vi "Init.vi"(8 "error in (no error)":errorcluster, 9 "Minimum Event Level":T1=enum."Info", 10 "EventLogger":refnum<class "EventLogHandler.lvclass">) -> (0 "error out":errorcluster, 3 "EventLoggingService out":refnum<class "EventLoggingService.lvclass">)   [LabVIEW 2020, in "Vecto.lvlib" / "EventLoggingService.lvclass"]
uses:
  EventLoggingService.lvclass
  EventLogHandler/EventLogHandler.lvclass
  Event Level.ctl
  EventLoggingService.lvclass/EventLoggingService.ctl
  <vilib>/Utility/error.llb/Error Cluster From Error Code.vi
  Vecto.lvlib
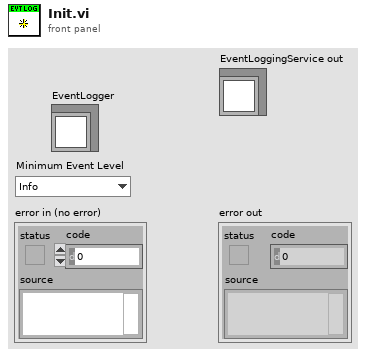
[diagram p1: front panel]
types:
  T1 = typedef "Vecto.lvlib/Event Level.ctl" = enum16{"Debug", "Info", "Warning", "Error"}
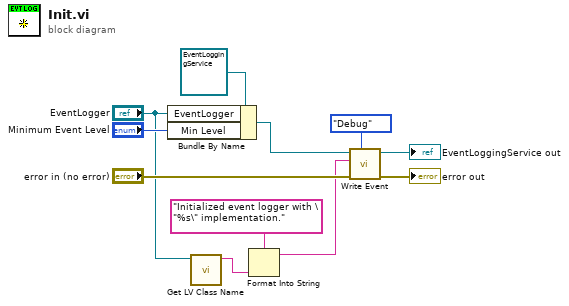
[diagram p0: block diagram]
diagram:
  n1 = Bundle By Name(cluster=refnum<class "EventLoggingService.lvclass"> refnum ("EventLoggingService in"), "EventLogger"="EventLogger", "Min Level"="Minimum Event Level") -> (w7:refnum<class "EventLoggingService.lvclass">)
  n2 = call <vilib>:"Get LV Class Name.vi"("object"="EventLogger") -> ("class name"=w3:string)  [unwired: 9 in, 1 out]
  n3 = Format Into String(format string="Initialized event logger with \"%s\" implementation.", w3) -> (resulting string=w1:string)  [unwired: 2 in, 1 out]
  n4 = call "Write Event.vi"("Event Level (Info)"=Event_Level."Debug", "error in (no error)"="error in (no error)", "Message"=w1, "EventLoggingService in"=w7) -> ("error out"=→"error out":errorcluster, "EventLoggingService out"=→"EventLoggingService out":refnum<class "EventLoggingService.lvclass">)  [unwired: 6 in]
